vi "CheckHu.vi"(1 "TargetTile":u16(ring)=36, 2 "Hand":u16[](array[ring])) -> (0 "CanHu":bool)   [LabVIEW 2025]
panel:
  out "HandCount":u16[](array[numeric])
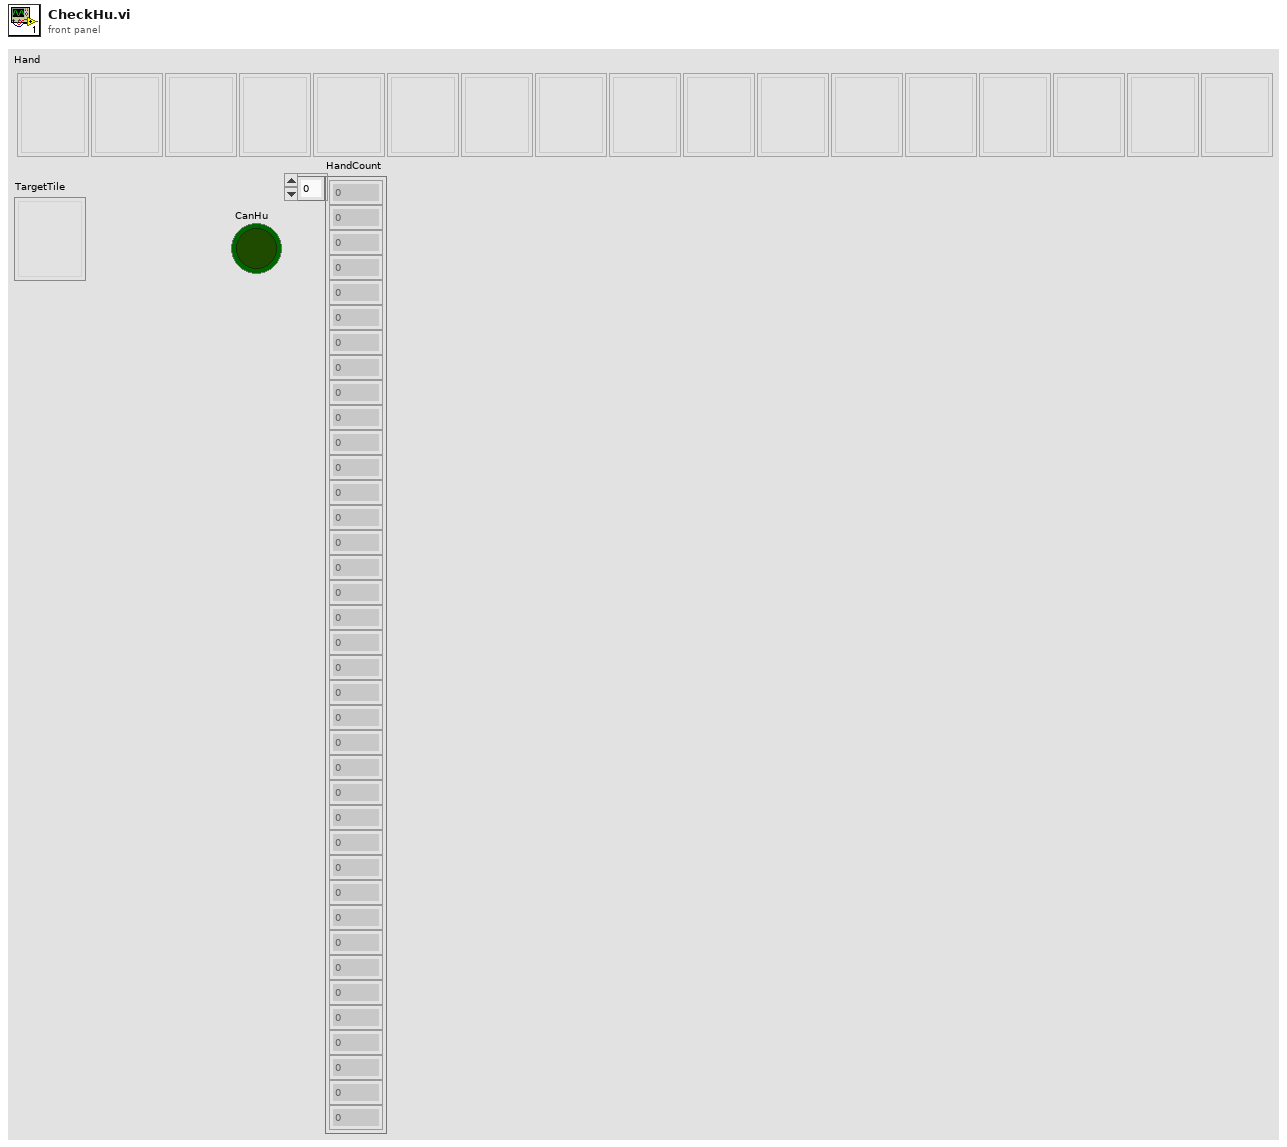
[diagram p1: front panel]
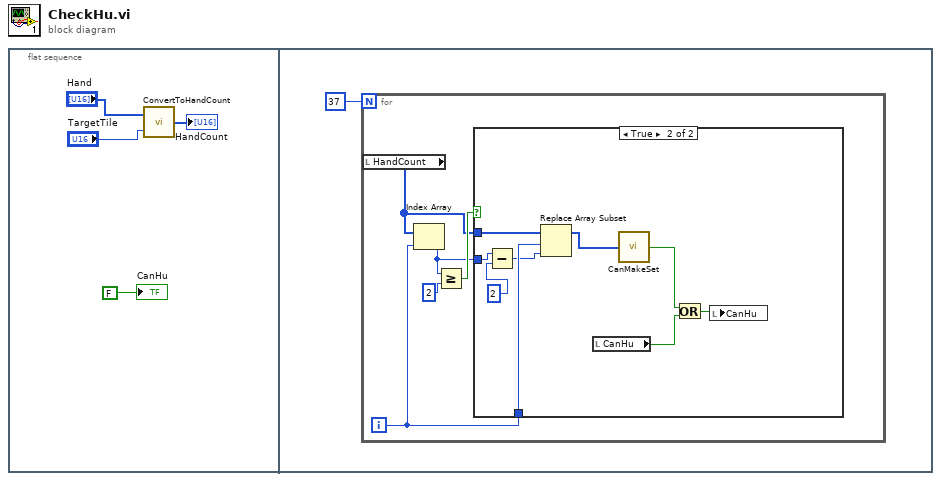
[diagram p0: block diagram]
diagram:
  n1 = flat-sequence {
    frame #0 {
      n2 = call "ConvertToHandCount.vi"("AddtionalTile"="TargetTile", "Hand"="Hand") -> ("HandCount"=→"HandCount":u16[])
      "CanHu" <- FALSE
    }
    frame #1 {
      n3 = for {
        N: 37 -> [_]
        i -> [w8]
        n4 = local read "HandCount"() -> (w7:u16[])
        n5 = Index Array(array=w7, index=w8) -> (element=w6:u16)
        n6 = Greater Or Equal?(x=w6, y=2) -> (x >= y?=w10:bool)
        n7 = case shown="True" w10 {
          tunnel: w8 -> [_ w19]
          tunnel: w7 -> [_ w18]
          tunnel: w6 -> [_ w16]
          frame False {
          }
          frame True {
            n8 = Subtract(x=w16, y=2) -> (x-y=w17:i32)
            n9 = Replace Array Subset(array=w18, new element=w17, index=w19) -> (w14:u16[])
            n10 = local read "CanHu"() -> (w12:bool)
            n11 = call "CanMakeSet.vi"("HandCount"=w14) -> ("CanMakeSet"=w11:bool)
            n12 = Or(x=w11, y=w12) -> (x .or. y?=w13:bool)
            n13 = local write "CanHu"(w13) -> ()
          }
        }
      }
    }
  }
